vi "Status Get Fault Status.vi"(0 "VISA resource name":refnum<visa-resource-name>, 2 "Retry Attempts (0)":i32 min=0, 11 "error in (no error)":errorcluster) -> (4 "VISA resource name out":refnum<visa-resource-name>, 6 "Upper Pressure Fault":bool, 8 "Lower Pressure Fault":bool, 10 "Motor Stall Fault":bool, 15 "error out":errorcluster)   [LabVIEW 2020, in "ChromTech Series III Pump.lvlib"]
doc: "Query the instrument for any current faults."
uses:
  ChromTech Series III Pump.lvlib
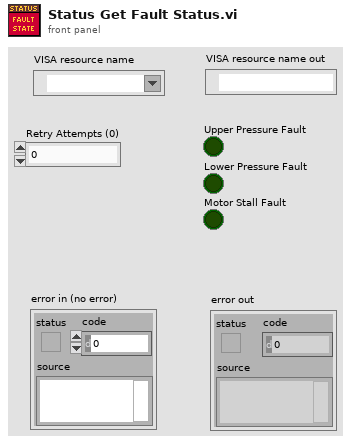
[diagram p1: front panel]
types:
  T1 = cluster{"Upper Pressure Fault":bool, "Lower Pressure Fault":bool, "Motor Stall Fault":bool}
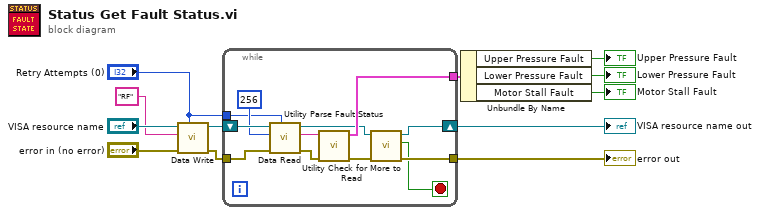
[diagram p0: block diagram]
diagram:
  n1 = call "Data Write.vi"("Retry Attempts (0)"="Retry Attempts (0)", "error in (no error)"="error in (no error)", "Command"="RF", "VISA Refnum in"="VISA resource name") -> ("error out"=w8:errorcluster, "VISA Refnum out"=w6:refnum<visa-resource-name>)  [unwired: 6 in]
  n2 = while {
    tunnel: [w18] -> w4
    shift-right: [w15] -> w2
    shift-left: w6 -> [w22]
    tunnel: "Retry Attempts (0)" -> [w13]
    tunnel: w8 -> [w24]
    tunnel: [w17] -> w3
    stop <- w14 stop-if-true
    n3 = call "Data Read.vi"("Retry Attempts (0)"=w13, "error in (no error)"=w24, "Bytes to read"=256, "VISA Refnum in"=w22) -> ("error out"=w23:errorcluster, "read buffer"=w19:string, "VISA Refnum out"=w16:refnum<visa-resource-name>)  [unwired: 5 in]
    n4 = call "Utility Parse Fault Status.vi"("error in (no error)"=w23, "Fault Status Response"=w19) -> ("error out"=w20:errorcluster, "Fault Status Cluster out"=w18:T1)  [unwired: 8 in]
    n5 = call "Utility Check for More to Read.vi"("error in (no error)"=w20, "VISA Refnum in"=w16) -> ("error out (unchanged)"=w17:errorcluster, "More to read?"=w14:bool, "VISA Refnum out"=w15:refnum<visa-resource-name>)  [unwired: 7 in]
  }
  "VISA resource name out" <- w2
  "error out" <- w3
  n6 = Unbundle By Name(w4) -> ("Upper Pressure Fault"=→"Upper Pressure Fault":bool, "Lower Pressure Fault"=→"Lower Pressure Fault":bool, "Motor Stall Fault"=→"Motor Stall Fault":bool)
